vi "play_verifyControlLaw.vi"() -> ()   [LabVIEW 2014]
uses:
  controls/controlParams_tracktraj.ctl
  <vilib>/FPGAPlugInAG/cRIO-9082/niLvFpga_Open_cRIO-9082.vi
  <vilib>/rvi/interface/common/dynamic/niFpgaDynamicAddResources.vi
  <vilib>/FPGAPlugInAG/Dynamic/niLvFpga_Reset_Dynamic.vi
  <vilib>/rvi/interface/common/niFpgaWaitOnOcc.vi
  <vilib>/Utility/error.llb/Error Cluster From Error Code.vi
  <vilib>/rvi/errors/niLvFpgaAdjustHostInterfaceError.vi
  <vilib>/FPGAPlugInAG/Dynamic/niLvFpga_Run_Dynamic.vi
  <vilib>/FPGAPlugInAG/Dynamic/niLvFpga_Close_Dynamic.vi
  <vilib>/rvi/interface/nirviOpenFPGA/nirviOpenFPGA.xnode
  FPGA Bitfiles/AFMsssinglematri_FPGATargetSPARTA_verifycontrolLaw_7X4CJNoWOHU.lvbitx
  FPGA Bitfiles/verify_controlLaw.vi
  <vilib>/rvi/interface/nirviMethod/nirviMethod.xnode
  <vilib>/rvi/interface/nirviReadWriteControl/nirviReadWriteControl.xnode
  <vilib>/rvi/interface/nirviCloseFPGA/nirviCloseFPGA.xnode
  <vilib>/rvi/errors/niLvFpgaMergeErrorWithErrorCode.vi
  <vilib>/rvi/interface/Simulation/niFpgaSimulationCallBeginRW.vi
  <vilib>/FPGAPlugInAG/Dynamic/niLvFpga_ConfigureFifo_Dynamic.vi
  <vilib>/FPGAPlugInAG/Dynamic/niLvFpga_WriteFifo_Dynamic.vi
  NiFpgaLv.dll
panel:
  in  "Ki":dbl format="%#_13g"
  in  "u_Kx_ref(k)":sgl
  in  "y_ref(k)":sgl
  in  "y(k) (from plant)":sgl
  in  "Xd_in":sgl[](array[numeric])=[0.0, 0.0, 0.0, 0.0, 0.0, 0.0, 0.0, 0.0, 0.0, 0.0, 0.0, 0.0]
  in  "x^(k)":sgl[](array[numeric])=[0.0, 0.0, 0.0, 0.0, 0.0, 0.0, 0.0, 0.0, 0.0, 0.0, 0.0, 0.0, 0.0, 0.0, 0.0, 0.0, 0.0, 0.0, 0.0, 0.0, 0.0, 0.0, 0.0, 0.0, 0.0]
  out "u(k) (saturated)":sgl
  out "x^(k+1) = Ax + Bu + Lye":sgl[](array[numeric])
  out "Xd_out(k+1)":sgl[](array[numeric])
  in  "umax":dbl=1.0 format="%#_13g"
  in  "Cluster 2":T1={"umax"=3.0, "y_ref(k)"=0.0, "Ki"=0.0, "y(k) (from plant)"=0.0, "ND"=0, "NS"=0, "u_Kx_ref(k)"=0.0} {"u_Kx_ref(k)" format="%#_13g"; "Ki" format="%#_13g"; "y_ref(k)" format="%#_13g"; "umax" format="%#_13g"}
  in  "Control Parameters path":path=path "C:/Users/arnold/Documents/MATLAB/AFM_SS/data/exp01Controls.csv"
  in  "Boolean":bool=TRUE
  out "Iter":i32
  out "error constant":errorcluster
  out "Depth":i32
  out "Elements Remaing":i32
  out "NS":i32
  out "Nd":i32
  out "output array":dbl[](array[numeric])
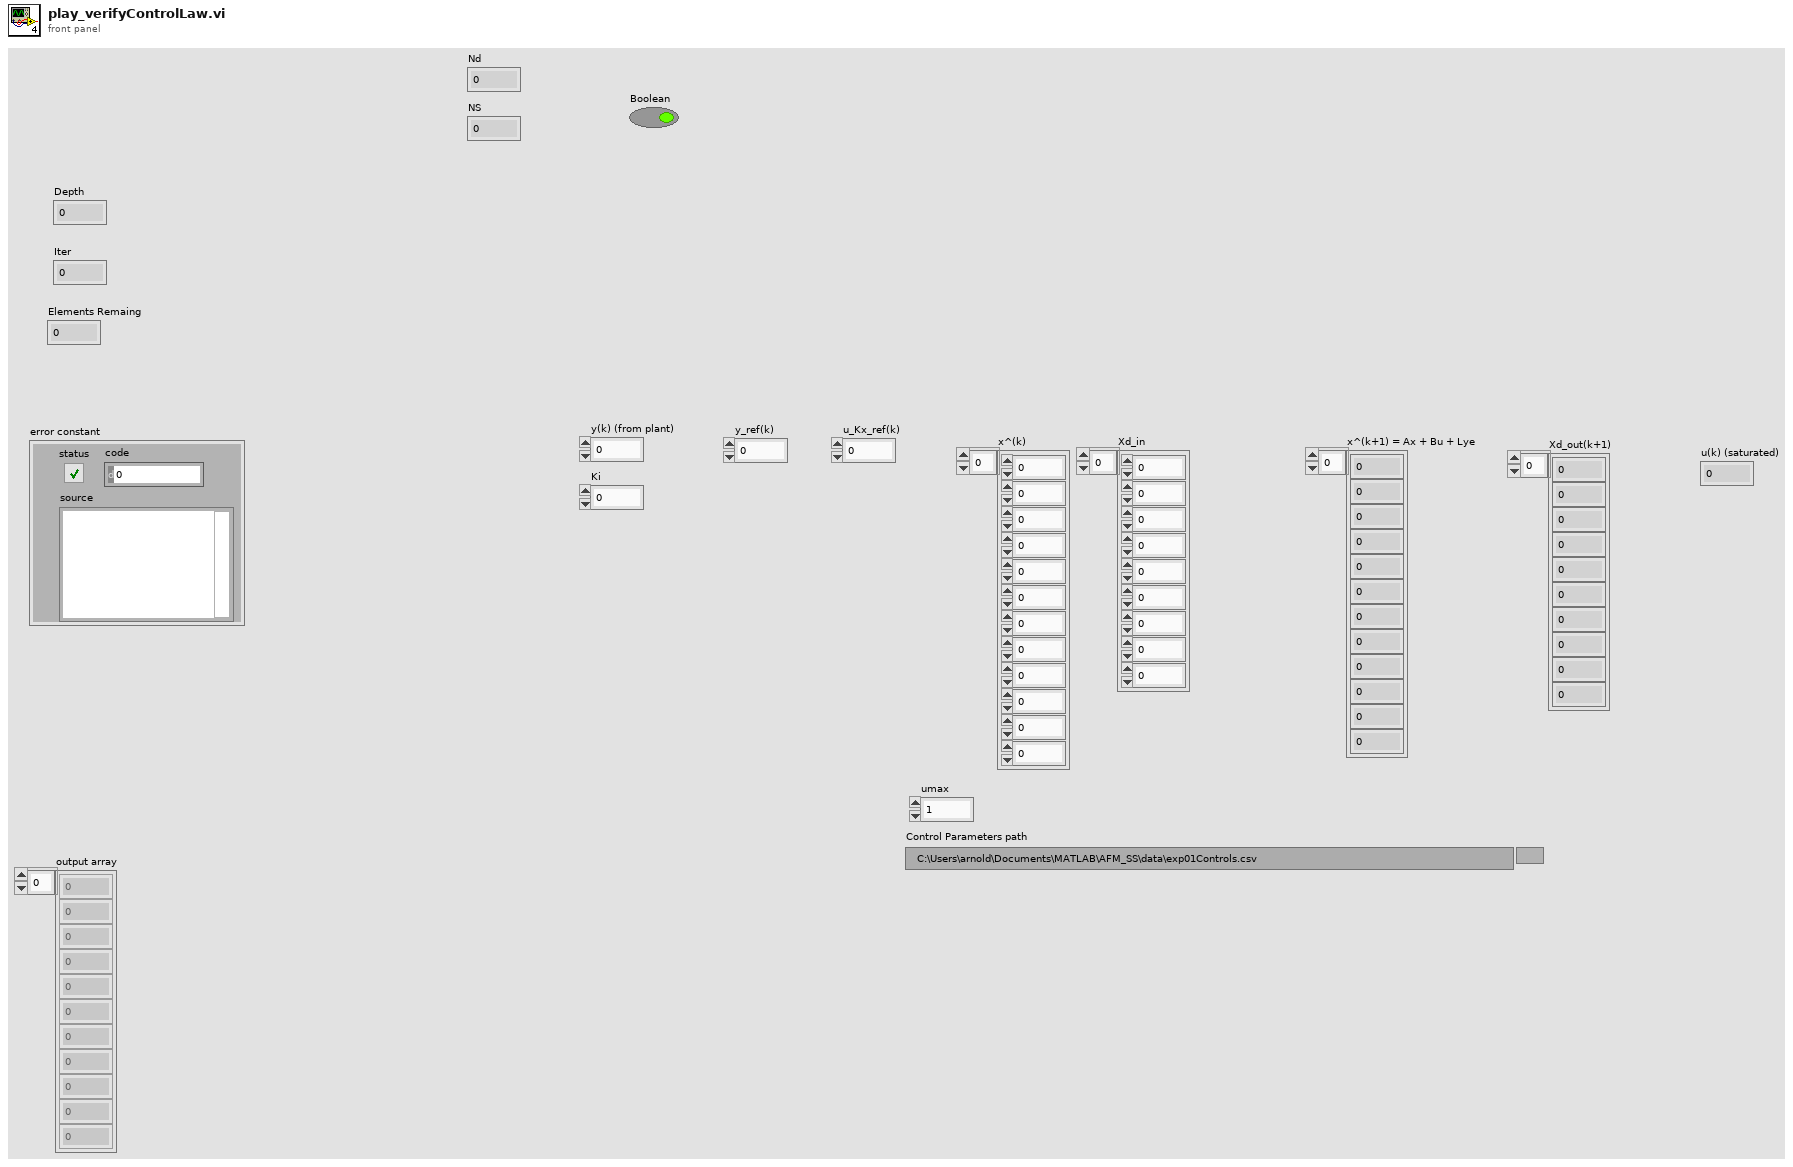
[diagram p1: front panel]
types:
  T1 = typedef "controlParams_tracktraj.ctl" = cluster{"umax":sgl, "y_ref(k)":sgl, "Ki":sgl, "y(k) (from plant)":sgl, "ND":i16, "NS":i16, "u_Kx_ref(k)":sgl}
  T2 = typedef "ControlParams.ctl" = cluster{"NS":i32, "ND":i32, "Nbar":dbl, "Ki":dbl, "ref":dbl}
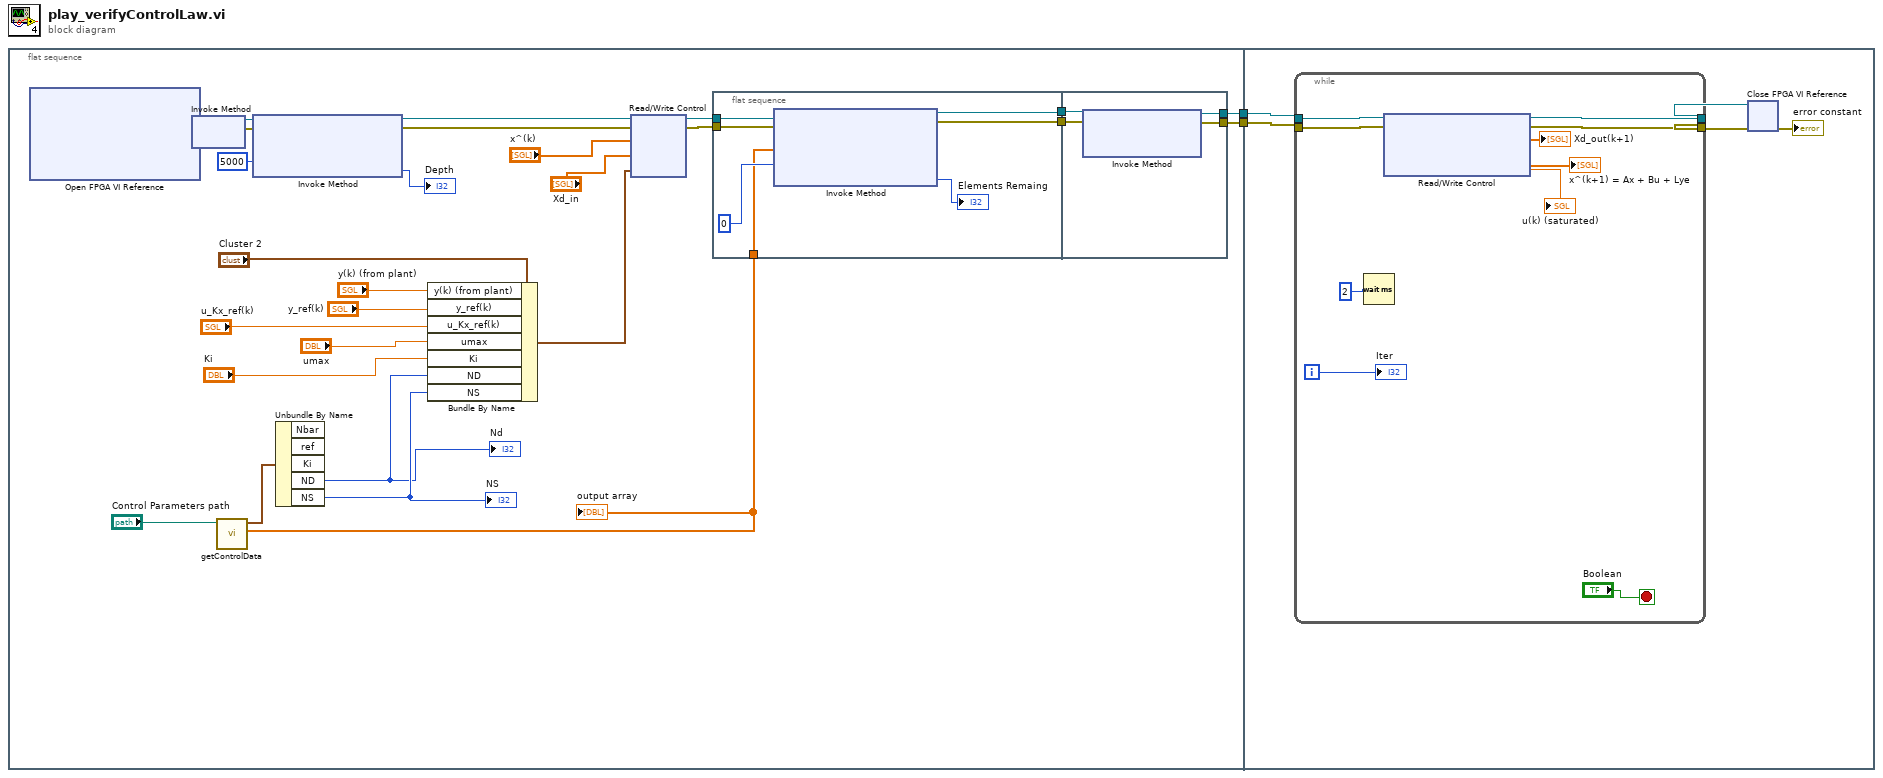
[diagram p0: block diagram]
diagram:
  n1 = flat-sequence {
    tunnel: [w22] -> w2
    tunnel: [w21] -> w1
    tunnel: w2 -> [w45]
    tunnel: w1 -> [w44]
    frame #0 {
      n2 = xnode "Open FPGA VI Reference"() -> ("FPGA VI Reference Out"=w26:refnum<k20>, "error out"=w27:errorcluster)  [unwired: 2 in]
      n3 = xnode "Invoke Method"("FPGA VI Reference In"=w26, "error in"=w27) -> ("FPGA VI Reference Out"=w29:refnum<k20>, "error out"=w30:errorcluster)
      n4 = call "getControlData.vi"("system matricec path"="Control Parameters path") -> ("AllMatrix"=w12:dbl[], "controlParams"=w14:T2)  [unwired: 9 in]
      "output array" <- w12
      n5 = xnode "Invoke Method"("FPGA VI Reference In"=w29, "error in"=w30, "Requested Depth"=5000) -> ("FPGA VI Reference Out"=w20:refnum<k20>, "error out"=w19:errorcluster, "Actual Depth"=→"Depth":u32)
      n6 = Unbundle By Name(w14) -> ("ND"=w4:i32, "NS"=w11:i32)  [unwired: 3 out]
      "NS" <- w11
      "Nd" <- w4
      n7 = Bundle By Name(cluster="Cluster 2", "y(k) (from plant)"="y(k) (from plant)", "y_ref(k)"="y_ref(k)", "u_Kx_ref(k)"="u_Kx_ref(k)", "umax"="umax", "Ki"="Ki", "ND"=w4, "NS"=w11) -> (w3:T1)
      n8 = xnode "Read/Write Control"("FPGA VI Reference In"=w20, "error in"=w19, "x^(k)"="x^(k)", "Xd_in"="Xd_in", "Cluster"=w3) -> ("FPGA VI Reference Out"=w24:refnum<k20>, "error out"=w23:errorcluster)
      n9 = flat-sequence {
        tunnel: w12 -> [w36]
        tunnel: w24 -> [w35]
        tunnel: w23 -> [w34]
        tunnel: [w33] -> w18
        tunnel: [w32] -> w17
        tunnel: w18 -> [w41]
        tunnel: w17 -> [w40]
        tunnel: [w39] -> w22
        tunnel: [w38] -> w21
        frame #0 {
          n10 = xnode "Invoke Method"("FPGA VI Reference In"=w35, "error in"=w34, "Data"=w36, "Timeout (ms)"=0) -> ("FPGA VI Reference Out"=w33:refnum<k20>, "error out"=w32:errorcluster, "Empty Elements Remaining"=→"Elements Remaing":u32)
        }
        frame #1 {
          n11 = xnode "Invoke Method"("FPGA VI Reference In"=w41, "error in"=w40) -> ("FPGA VI Reference Out"=w39:refnum<k20>, "error out"=w38:errorcluster)  [unwired: 1 in]
        }
      }
    }
    frame #1 {
      n12 = while {
        tunnel: [w51] -> w42
        tunnel: [w50] -> w43
        tunnel: w45 -> [w53]
        tunnel: w44 -> [w52]
        i -> [w56]
        stop <- "Boolean" stop-if-true
        n13 = Wait (ms)(milliseconds to wait=2) -> ()  [unwired: 1 out]
        n14 = xnode "Read/Write Control"("FPGA VI Reference In"=w53, "error in"=w52) -> ("FPGA VI Reference Out"=w51:refnum<k20>, "error out"=w50:errorcluster, "Xd_out(k+1)"=→"Xd_out(k+1)":sgl[], "x^(k+1) = Ax + Bu + Lye"=→"x^(k+1) = Ax + Bu + Lye":sgl[], "u(k) (saturated)"=→"u(k) (saturated)":sgl)
        "Iter" <- w56
      }
      n15 = xnode "Close FPGA VI Reference"("FPGA VI Reference In"=w42, "error in"=w43) -> ("error out"=→"error constant":errorcluster)
    }
  }
